vi "GUI_Encoder.vi"() -> ()   [LabVIEW 2013]
uses:
  <vilib>/Instr/_visa.llb/VISA Configure Serial Port (Instr).vi
panel:
  in  "Angle":u16
  in  "OK":bool
  in  "Commands":string(combo)
  in  "Stop":bool
  out "error out 2":errorcluster
  in  "Baud Rate":u32=9600
  in  "Port":refnum<visa-resource-name>
  out "Response":string
  in  "MODE":bool
  out "error out":errorcluster
  out "Response":string
  in  "Command":string
  # "Encoder Interface"
  # "Text Mode"
  # "Select : ON : Text Mode , \n              OFF : ButtonMode"
  # "Button Mode"
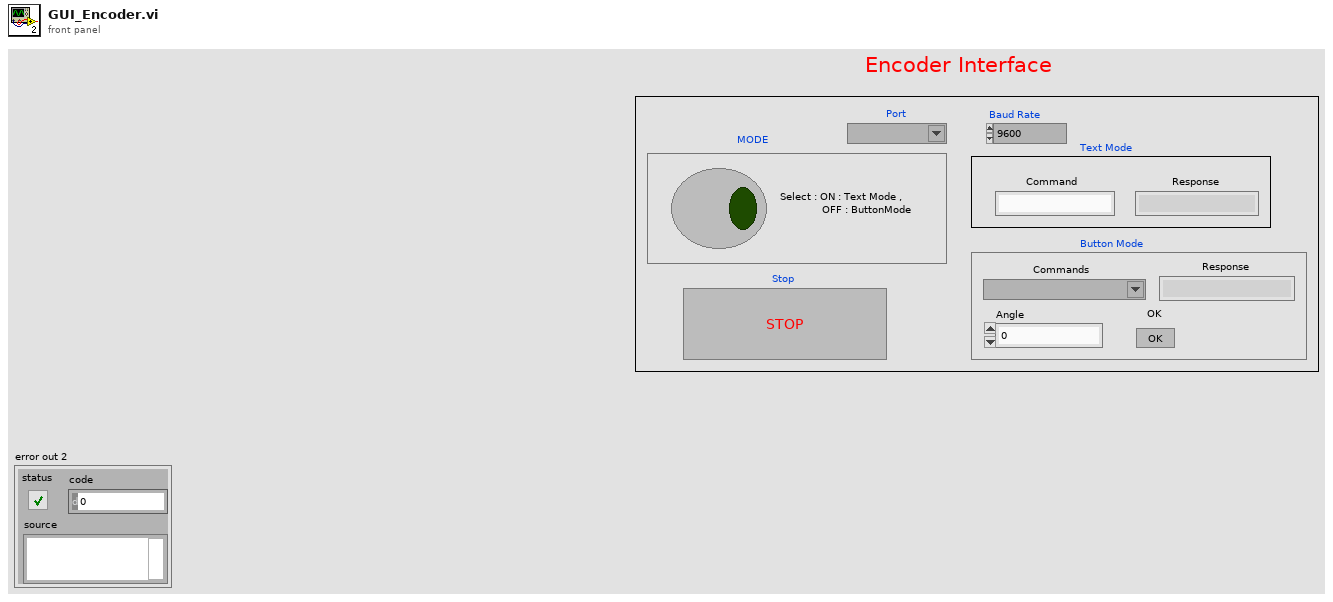
[diagram p1: front panel]
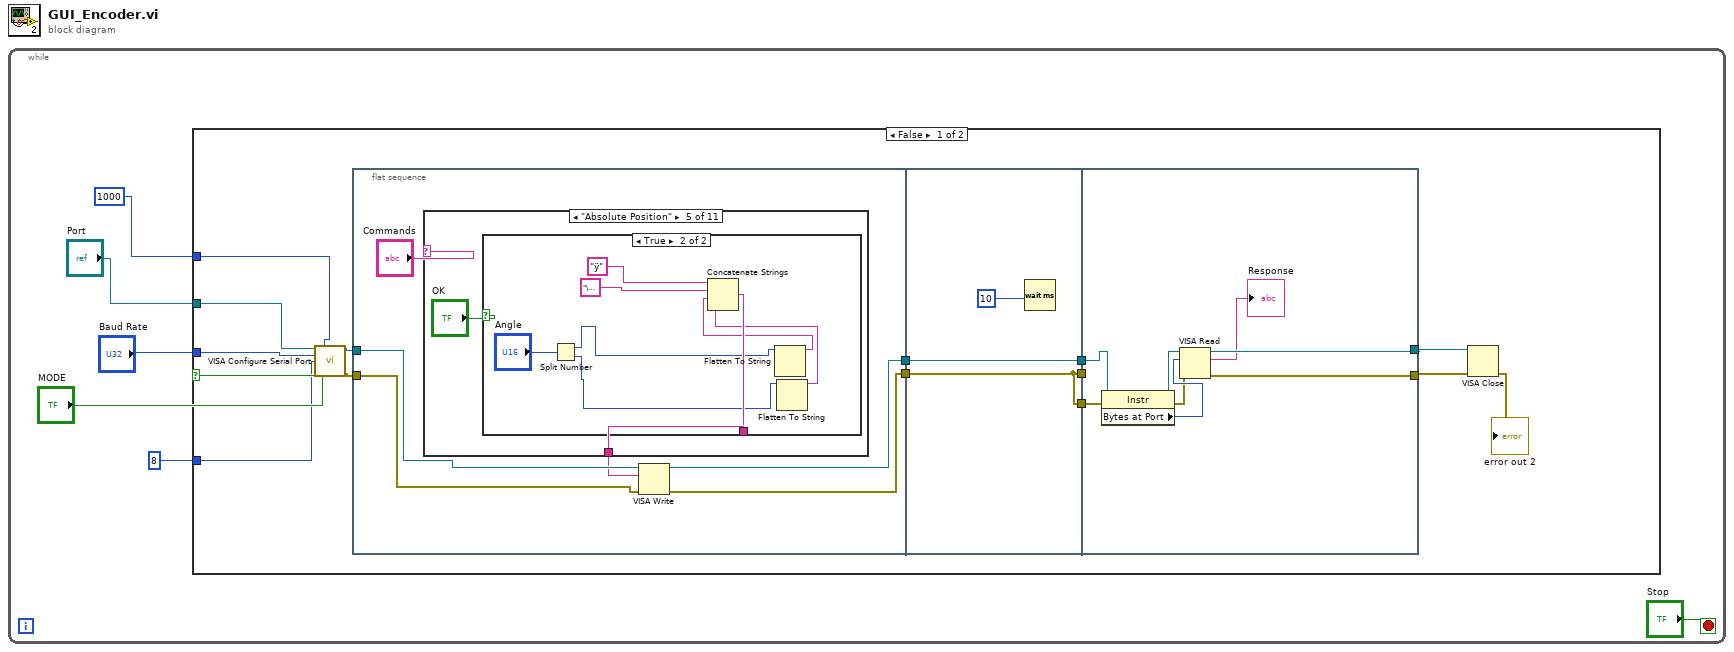
[diagram p0: block diagram]
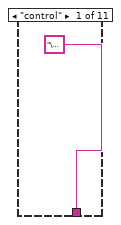
[diagram p2: hidden frame]
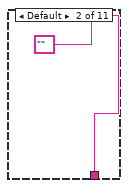
[diagram p3: hidden frame]
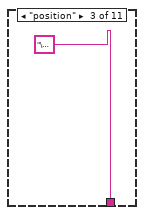
[diagram p4: hidden frame]
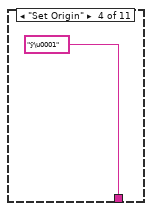
[diagram p5: hidden frame]
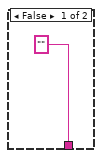
[diagram p6: hidden frame]
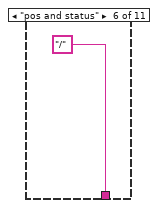
[diagram p7: hidden frame]
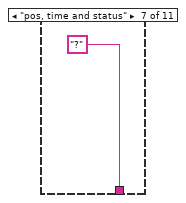
[diagram p8: hidden frame]
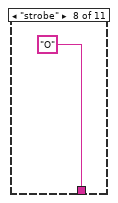
[diagram p9: hidden frame]
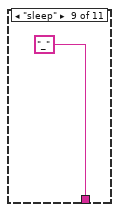
[diagram p10: hidden frame]
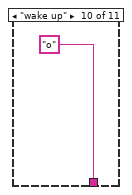
[diagram p11: hidden frame]
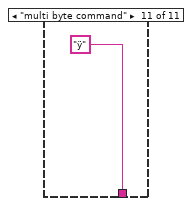
[diagram p12: hidden frame]
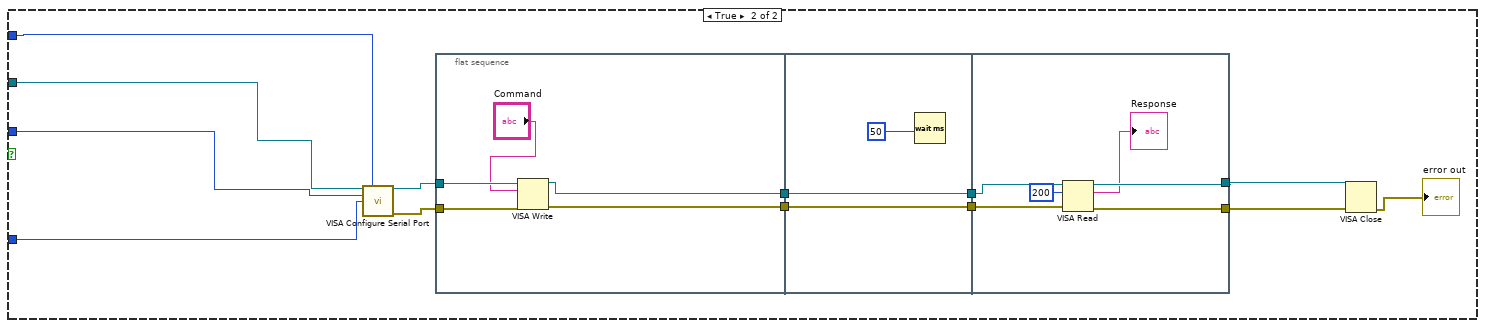
[diagram p13: hidden frame]
diagram:
  n1 = while {
    stop <- "Stop" stop-if-true
    n2 = case shown="False" "MODE" {
      tunnel: u32 1000 ("timeout (10sec)") -> [w10 w62]
      tunnel: "Port" -> [w9 w61]
      tunnel: "Baud Rate" -> [w8 w60]
      tunnel: u16 8 ("data bits (8)") -> [w7 w59]
      frame False {
        n3 = call-poly "VISA Configure Serial Port"("VISA resource name"=w9, "timeout (10sec)"=w10, "baud rate (9600)"=w8, "data bits (8)"=w7) -> ("VISA resource name out"=w16:refnum<visa-resource-name>, "error out"=w15:errorcluster)  [unwired: 10 in]
        n4 = flat-sequence {
          tunnel: [w25] -> w20
          tunnel: w16 -> [w24]
          tunnel: w15 -> [w23]
          tunnel: [w26] -> w14
          tunnel: [w49] -> w19
          tunnel: [w48] -> w18
          tunnel: w20 -> [w48]
          tunnel: w14 -> [w49]
          tunnel: [w48] -> w11
          tunnel: w19 -> [w54]
          tunnel: w18 -> [_]
          tunnel: [w58] -> w12
          tunnel: [w57] -> w13
          tunnel: w11 -> [w53]
          frame #0 {
            n5 = case shown="\"Absolute Position\"" "Commands" {
              tunnel: ["\u000f" "" "\u001f" "ÿ\u0001" w32 "/" "?" "O" "_" "o" "ÿ"] -> w21
              frame "control" {
              }
              frame Default {
              }
              frame "position" {
              }
              frame "Set Origin" {
              }
              frame "Absolute Position" {
                n6 = case shown="True" "OK" {
                  tunnel: ["" w39] -> w32
                  frame False {
                  }
                  frame True {
                    n7 = Split Number(x="Angle") -> (hi(x)=w37:u8, lo(x)=w35:u8)
                    n8 = Flatten To String(anything=w37) -> (data string=w36:string)  [unwired: 3 in, 2 out]
                    n9 = Flatten To String(anything=w35) -> (data string=w34:string)  [unwired: 3 in, 2 out]
                    n10 = Concatenate Strings("ÿ" ("string"), "\u0002" ("string"), w36, w34) -> (w39:string)
                  }
                }
              }
              frame "pos and status" {
              }
              frame "pos, time and status" {
              }
              frame "strobe" {
              }
              frame "sleep" {
              }
              frame "wake up" {
              }
              frame "multi byte command" {
              }
            }
            n11 = VISA Write(VISA resource name=w24, write buffer=w21, error in (no error)=w23) -> (VISA resource name out=w26:refnum<visa-resource-name>, error out=w25:errorcluster)  [unwired: 1 out]
          }
          frame #1 {
            n12 = Wait (ms)(milliseconds to wait=u32 10) -> ()  [unwired: 1 out]
          }
          frame #2 {
            n13 = property class="Instr"(reference=w54, error in=w53) -> (reference out=w52:refnum<visa-resource-name>, error out=w51:errorcluster, "Bytes at Port"=w55:u32)
            n14 = VISA Read(VISA resource name=w52, byte count=w55, error in (no error)=w51) -> (VISA resource name out=w57:refnum<visa-resource-name>, read buffer=→"Response":string, error out=w58:errorcluster)  [unwired: 1 out]
          }
        }
        n15 = VISA Close(VISA resource name=w13, error in (no error)=w12) -> (error out=→"error out 2":errorcluster)
      }
      frame True {
        n16 = call-poly "VISA Configure Serial Port"("VISA resource name"=w61, "timeout (10sec)"=w62, "baud rate (9600)"=w60, "data bits (8)"=w59) -> ("VISA resource name out"=w67:refnum<visa-resource-name>, "error out"=w66:errorcluster)  [unwired: 10 in]
        n17 = flat-sequence {
          tunnel: w67 -> [w74]
          tunnel: w66 -> [w76]
          tunnel: [w73] -> w71
          tunnel: [w75] -> w70
          tunnel: [w78] -> w69
          tunnel: w71 -> [w78]
          tunnel: [w77] -> w68
          tunnel: w70 -> [w77]
          tunnel: w69 -> [w85]
          tunnel: w68 -> [w84]
          tunnel: [w83] -> w64
          tunnel: [w82] -> w65
          frame #0 {
            n18 = VISA Write(VISA resource name=w74, write buffer="Command", error in (no error)=w76) -> (VISA resource name out=w73:refnum<visa-resource-name>, error out=w75:errorcluster)  [unwired: 1 out]
          }
          frame #1 {
            n19 = Wait (ms)(milliseconds to wait=u32 50) -> ()  [unwired: 1 out]
          }
          frame #2 {
            n20 = VISA Read(VISA resource name=w85, byte count=u32 200, error in (no error)=w84) -> (VISA resource name out=w82:refnum<visa-resource-name>, read buffer=→"Response":string, error out=w83:errorcluster)  [unwired: 1 out]
          }
        }
        n21 = VISA Close(VISA resource name=w65, error in (no error)=w64) -> (error out=→"error out":errorcluster)
      }
    }
  }
